vi "GetFeaturesForMCSA(HandL).vi"(6 "supported metrics":string[](array[string]), 8 "error in (no error)":errorcluster, 9 "Metric Cache":variant, 11 "ChannelModel":T5) -> (0 "error out":errorcluster, 2 "channel":T1)   [LabVIEW 2017, in "McsaAnalysisFunctions.lvlib"]
uses:
  <vilib>/addons/InsightCM/Utilities/Analysis/MCSA/McsaAnalysisFunctions.lvlib
  <vilib>/addons/InsightCM/MessageBus/Base/controls/R2_Channel.ctl
  <vilib>/addons/InsightCM/MessageBus/Base/controls/KeyValuePair.ctl
  <vilib>/addons/InsightCM/MessageBus/Base/controls/Metric.ctl
  <vilib>/addons/InsightCM/Utilities/Analysis/MCSA/controls/McsaChannel.ctl
  <vilib>/addons/InsightCM/Utilities/Analysis/Shared/controls/Feature.ctl
  <vilib>/addons/InsightCM/Utilities/Analysis/Shared/controls/AmplitudeScale.ctl
  <vilib>/addons/InsightCM/Utilities/Analysis/Shared/AnalysisHelper.lvlib
  <vilib>/addons/InsightCM/Utilities/Tdms/Tdms.lvlib
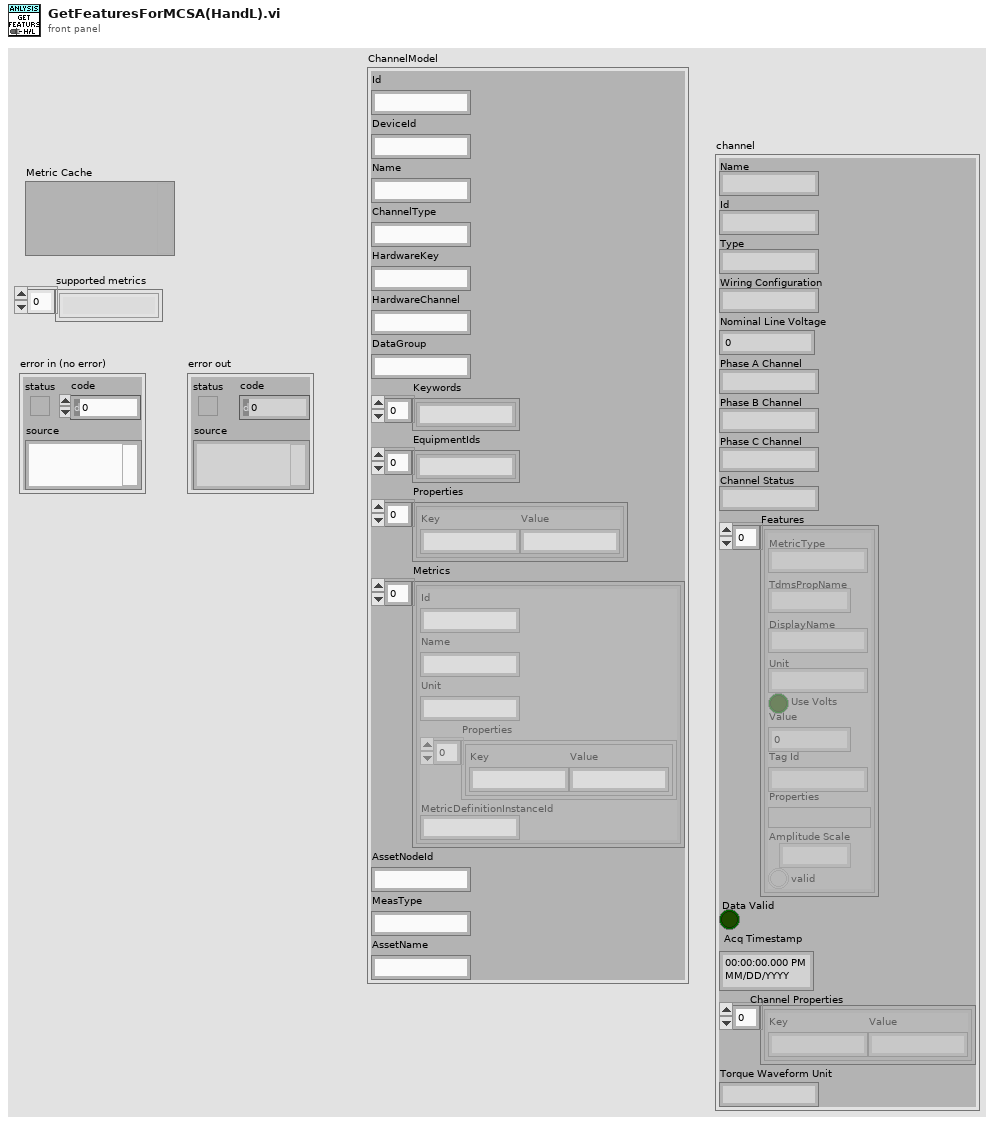
[diagram p1: front panel]
types:
  T1 = typedef "McsaAnalysisFunctions.lvlib/McsaChannel.ctl" = cluster{"Name":string, "Id":string, "Type":string, "Wiring Configuration":string, "Nominal Line Voltage":dbl, "Phase A Channel":string, "Phase B Channel":string, "Phase C Channel":string, "Channel Status":string, "Features":T2[], "Data Valid":bool, "Acq Timestamp":timestamp, "Channel Properties":T4[], "Torque Waveform Unit":string}
  T2 = typedef "AnalysisHelper.lvlib/Feature.ctl" = cluster{"MetricType":string, "TdmsPropName":string, "DisplayName":string, "Unit":string, "Use Volts":bool, "Value":dbl, "Tag Id":string, "Properties":variant, "Amplitude Scale":T3, "valid":bool}
  T3 = typedef "AnalysisHelper.lvlib/AmplitudeScale.ctl" = enum16{"rms", "peak", "pk-pk"}
  T4 = typedef "KeyValuePair.ctl" = cluster{"Key":string, "Value":string}
  T5 = typedef "R2_Channel.ctl" = cluster{"Id":string, "DeviceId":string, "Name":string, "ChannelType":string, "HardwareKey":string, "HardwareChannel":string, "DataGroup":string, "Keywords":string[], "EquipmentIds":string[], "Properties":T4[], "Metrics":T6[], "AssetNodeId":string, "MeasType":string, "AssetName":string}
  T6 = typedef "Metric.ctl" = cluster{"Id":string, "Name":string, "Unit":string, "Properties":T4[], "MetricDefinitionInstanceId":string}
  T7 = typedef "AnalysisHelper.lvlib/BandConfig.ctl" = cluster{"High":dbl, "Low":dbl, "Domain":T8, "Calculation":T9}
  T8 = typedef "AnalysisHelper.lvlib/BandDomain.ctl" = enum16{"Frequency", "CPM", "Orders"}
  T9 = typedef "AnalysisHelper.lvlib/BandCalculation.ctl" = enum16{"Total", "Max", "Phase"}
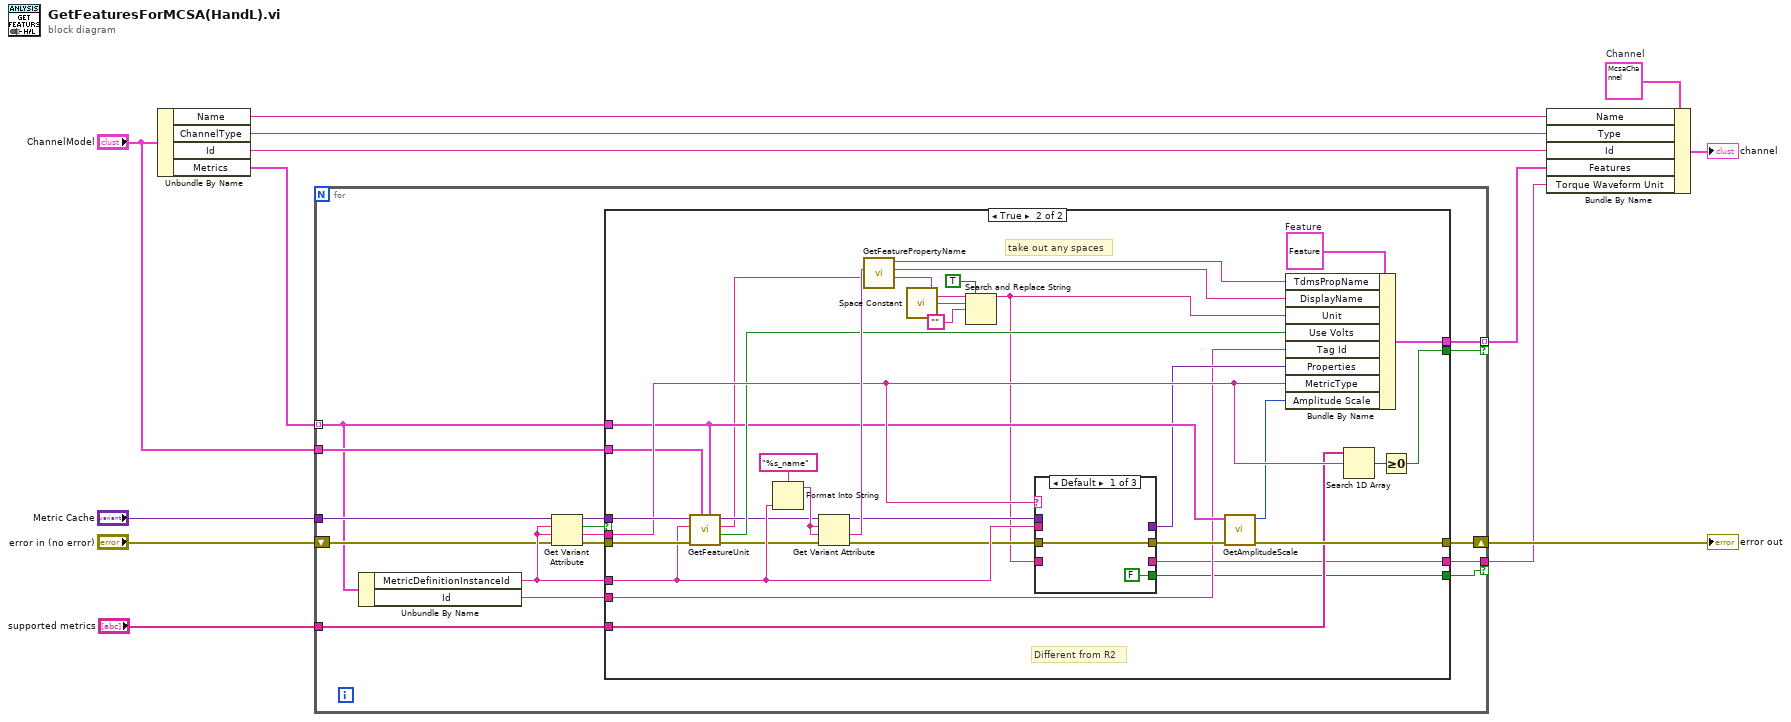
[diagram p0: block diagram]
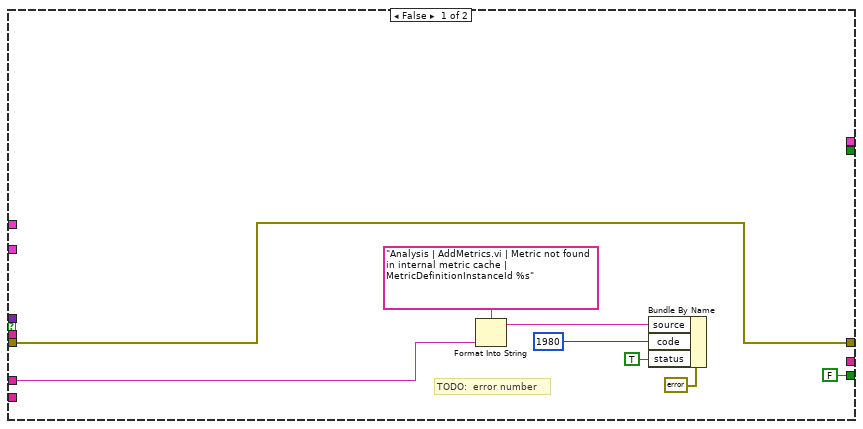
[diagram p2: hidden frame]
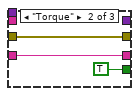
[diagram p3: hidden frame]
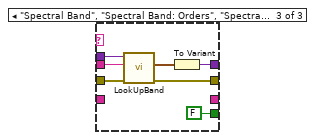
[diagram p4: hidden frame]
diagram:
  w2 = T1 {"Name"="", "Id"="", "Type"="", "Wiring Configuration"="", "Nominal Line Voltage"=0.0, "Phase A Channel"="", "Phase B Channel"="", "Phase C Channel"="", "Channel Status"="", "Features"=[], "Data Valid"=FALSE, "Acq Timestamp"=timestamp(0 s since 1904-01-01), "Channel Properties"=[], "Torque Waveform Unit"=""}  # Channel
  n1 = Unbundle By Name("ChannelModel") -> ("Name"=w4:string, "ChannelType"=w8:string, "Id"=w9:string, "Metrics"=w11:T6[])
  n2 = for {
    tunnel: "Metric Cache" -> [w19]
    tunnel: w11 -> [w17] mode=indexing
    tunnel: [w24] -> w10 mode=indexing if=w23
    shift-right: [w25] -> w6
    shift-left: "error in (no error)" -> [w20]
    tunnel: "ChannelModel" -> [w18]
    tunnel: "supported metrics" -> [w16]
    tunnel: [w15] -> w1 if=w14
    n3 = Unbundle By Name(w17) -> ("MetricDefinitionInstanceId"=w21:string, "Id"=w22:string)
    n4 = Get Variant Attribute(Variant=w19, name=w21, default value (empty Variant)=w21, error in=w20) -> (duplicate Variant=w26:variant, found=w27:bool, value=w29:string, error out=w28:errorcluster)
    n5 = case shown="True" w27 {
      tunnel: w28 -> [w31 w64]
      tunnel: w29 -> [_ w62]
      tunnel: w22 -> [_ w42]
      tunnel: w26 -> [_ w63]
      tunnel: [w31 w54] -> w25
      tunnel: [_ w68] -> w24
      tunnel: [_ w60] -> w23
      tunnel: w21 -> [w32 w59]
      tunnel: w17 -> [_ w53]
      tunnel: w18 -> [_ w58]
      tunnel: w16 -> [_ w43]
      tunnel: [_ w39] -> w15
      tunnel: [FALSE w38] -> w14
      frame False {
        # "TODO:  error number"
        n6 = Format Into String(format string="Analysis | AddMetrics.vi | Metric not found in internal metric cache | MetricDefinitionInstanceId %s" ("source"), w32) -> (resulting string=w35:string)  [unwired: 2 in, 1 out]
        n7 = Bundle By Name(cluster=errorcluster {"status"=FALSE, "code"=0, "source"=""} ("error out"), "source"=w35, "code"=1980, "status"=TRUE) -> ()  [unwired: 1 out]
      }
      frame True {
        w71 = T2 {"MetricType"="", "TdmsPropName"="", "DisplayName"="", "Unit"="", "Use Volts"=FALSE, "Value"=0.0, "Tag Id"="", "Properties"=variant(string ""), "Amplitude Scale"=enum."rms", "valid"=FALSE}  # Feature
        # "Different from R2"
        # "take out any spaces"
        n8 = call <vilib>:"GetFeatureUnit.vi"("metric"=w53, "channel"=w58, "error in (no error)"=w64, "metric definitionInstance id"=w59, "metric cache in"=w63) -> ("error out"=w55:errorcluster, "use volts"=w57:bool, "unit"=w48:string, "metric cache out"=w56:variant)  [unwired: 3 in]
        n9 = Format Into String(format string="%s_name", w59) -> (resulting string=w69:string)  [unwired: 2 in, 1 out]
        n10 = Get Variant Attribute(Variant=w56, name=w69, default value (empty Variant)=w69, error in=w55) -> (duplicate Variant=w46:variant, value=w66:string, error out=w41:errorcluster)  [unwired: 1 out]
        n11 = call <vilib>:"GetFeaturePropertyName.vi"("unit"=w48, "metric name"=w66) -> ("tdms unit value"=w47:string, "display name"=w67:string, "tdms property name"=w65:string)  [unwired: 7 in]
        n12 = call <vilib>:"Space Constant.vi"() -> ("String"=w50:string)
        n13 = Search and Replace String(replace all?=TRUE ("replace all? (F)"), input string=w47, search string=w50, replace string="") -> (result string=w40:string)  [unwired: 4 in, 3 out]
        n14 = case shown="Default" w62 {
          tunnel: w46 -> [_ _ w83]
          tunnel: w41 -> [w73 w76 w82]
          tunnel: [_ _ w78] -> w45
          tunnel: w59 -> [_ _ w79]
          tunnel: [w73 w76 w80] -> w44
          tunnel: w40 -> [_ w75 _]
          tunnel: [_ w75 _] -> w39
          tunnel: [FALSE TRUE FALSE] -> w38
          frame Default {
          }
          frame "Torque" {
          }
          frame "Spectral Band", "Spectral Band: Orders", "Spectral Band: Phase" {
            n15 = call <vilib>:"LookUpBand.vi"("error in (no error)"=w82, "MetricDefinitionInstanceId"=w79, "Metric Cache"=w83) -> ("error out"=w80:errorcluster, "SpectralBand"=w81:T7)  [unwired: 6 in, 1 out]
            n16 = To Variant(anything=w81) -> (Variant=w78:variant)
          }
        }
        n17 = call <vilib>:"GetAmplitudeScale.vi"("error in (no error)"=w44, "metric"=w53) -> ("error out"=w54:errorcluster, "amplitude scale"=w52:T3)  [unwired: 8 in]
        n18 = Bundle By Name(cluster=w71, "TdmsPropName"=w65, "DisplayName"=w67, "Unit"=w40, "Use Volts"=w57, "Tag Id"=w42, "Properties"=w45, "MetricType"=w62, "Amplitude Scale"=w52) -> (w68:T2)
        n19 = Search 1D Array(1D array=w43, element=w62) -> (index of element=w61:i32)  [unwired: 1 in]
        n20 = Greater Or Equal To 0?(x=w61) -> (x >= 0?=w60:bool)
      }
    }
  }
  "error out" <- w6
  n21 = Bundle By Name(cluster=w2, "Name"=w4, "Type"=w8, "Id"=w9, "Features"=w10, "Torque Waveform Unit"=w1) -> (→"channel":T1)
